vi "E3631A_Voltage Controller.vi"(5 "Channel Controller":T1(ring)=enum."Voltage 3", 6 "Voltage 3":dbl=-3.3 format="%.3g", 7 "Initialize":bool, 8 "error in (no error)":errorcluster, 9 "Voltage 2":dbl=3.3 format="%.3g", 10 "Voltage 1":dbl=3.3 format="%.3g", 11 "VISA resource name":refnum<visa-resource-name>="GPIB0::5::INSTR") -> (0 "error out":errorcluster, 3 "VISA resource name out":refnum<visa-resource-name>="GPIB0::5::INSTR")   [LabVIEW 2012]
uses:
  _Employee_Folders/Andy temp/All Driver/agilent/Agilent E363X Series/Agilent E363X Series.lvlib
panel:
  in  "Channel 3":i32(ring)=3 items=["Channel 1"=1, "Channel 2"=2, "Channel 3"=3]
  in  "Channel 2":i32(ring)=2 items=["Channel 1"=1, "Channel 2"=2, "Channel 3"=3]
  in  "Channel 1":i32(ring)=1 items=["Channel 1"=1, "Channel 2"=2, "Channel 3"=3]
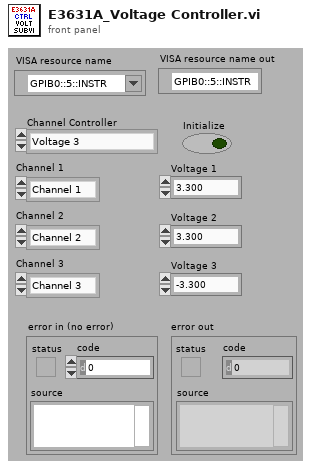
[diagram p1: front panel]
types:
  T1 = enum16{"Idle...", "Voltage 1", "Voltage 2", "Voltage 3"}
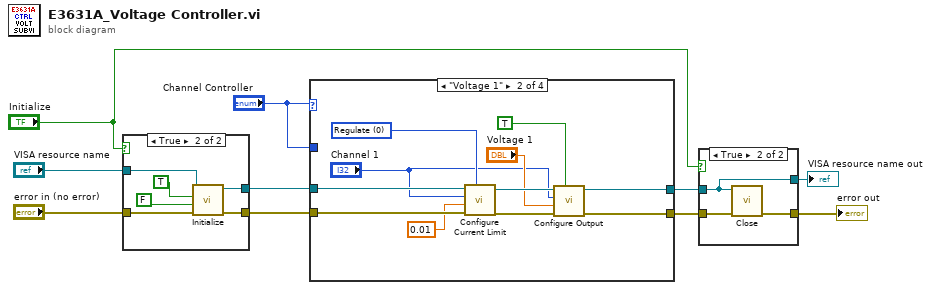
[diagram p0: block diagram]
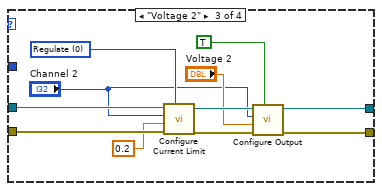
[diagram p5: hidden frame]
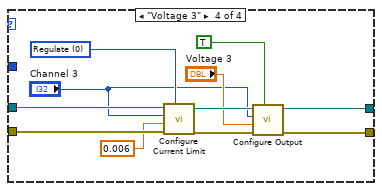
[diagram p6: hidden frame]
diagram:
  n1 = case shown="True" "Initialize" {
    tunnel: "error in (no error)" -> [w11 w18]
    tunnel: [w11 w17] -> w9
    tunnel: [w12 w16] -> w8
    tunnel: "VISA resource name" -> [w12 w13]
    frame False {
    }
    frame True {
      n2 = call "Initialize.vi"("error in (no error)"=w18, "Reset? (T: Yes)"=FALSE, "ID Query? (T: Yes)"=TRUE, "VISA resource name"=w13) -> ("error out"=w17:errorcluster, "VISA resource name out"=w16:refnum<visa-resource-name>)  [unwired: 6 in]
    }
  }
  n3 = case shown="\"Voltage 1\"" "Channel Controller" {
    tunnel: w9 -> [w19 w31 w42 w53]
    tunnel: w8 -> [w20 w30 w41 w52]
    tunnel: [w19 w24 w35 w46] -> w7
    tunnel: [w20 w23 w34 w45] -> w6
    tunnel: "Channel Controller" -> [_ _ _ _]
    frame "Idle...", Default {
    }
    frame "Voltage 1" {
      w28 = u16 0 items=["Regulate", "Trip"] ("Behavior (0: Regulate)")
      n4 = call "Configure Current Limit.vi"("Behavior (0: Regulate)"=w28, "error in (no error)"=w31, "Current Limit (0.0 A)"=0.01, "Channel (1: Channel 1)"="Channel 1", "VISA resource name"=w30) -> ("error out"=w26:errorcluster, "VISA resource name out"=w27:refnum<visa-resource-name>)  [unwired: 5 in]
      n5 = call "Configure Output.vi"("Enable Output (T: Enable)"=TRUE, "error in (no error)"=w26, "Voltage Level (0.0 V)"="Voltage 1", "Channel (1: Channel 1)"="Channel 1", "VISA resource name"=w27) -> ("error out"=w24:errorcluster, "VISA resource name out"=w23:refnum<visa-resource-name>)  [unwired: 5 in]
    }
    frame "Voltage 2" {
      w39 = u16 0 items=["Regulate", "Trip"] ("Behavior (0: Regulate)")
      n6 = call "Configure Current Limit.vi"("Behavior (0: Regulate)"=w39, "error in (no error)"=w42, "Current Limit (0.0 A)"=0.2, "Channel (1: Channel 1)"="Channel 2", "VISA resource name"=w41) -> ("error out"=w37:errorcluster, "VISA resource name out"=w38:refnum<visa-resource-name>)  [unwired: 5 in]
      n7 = call "Configure Output.vi"("Enable Output (T: Enable)"=TRUE, "error in (no error)"=w37, "Voltage Level (0.0 V)"="Voltage 2", "Channel (1: Channel 1)"="Channel 2", "VISA resource name"=w38) -> ("error out"=w35:errorcluster, "VISA resource name out"=w34:refnum<visa-resource-name>)  [unwired: 5 in]
    }
    frame "Voltage 3" {
      w50 = u16 0 items=["Regulate", "Trip"] ("Behavior (0: Regulate)")
      n8 = call "Configure Current Limit.vi"("Behavior (0: Regulate)"=w50, "error in (no error)"=w53, "Current Limit (0.0 A)"=0.006, "Channel (1: Channel 1)"="Channel 3", "VISA resource name"=w52) -> ("error out"=w48:errorcluster, "VISA resource name out"=w49:refnum<visa-resource-name>)  [unwired: 5 in]
      n9 = call "Configure Output.vi"("Enable Output (T: Enable)"=TRUE, "error in (no error)"=w48, "Voltage Level (0.0 V)"="Voltage 3", "Channel (1: Channel 1)"="Channel 3", "VISA resource name"=w49) -> ("error out"=w46:errorcluster, "VISA resource name out"=w45:refnum<visa-resource-name>)  [unwired: 5 in]
    }
  }
  n10 = case shown="True" "Initialize" {
    tunnel: w7 -> [w55 w58]
    tunnel: w6 -> [w54 w56]
    tunnel: [w55 w57] -> w5
    tunnel: [w54 w56] -> w1
    frame False {
    }
    frame True {
      n11 = call "Close.vi"("error in (no error)"=w58, "VISA resource name"=w56) -> ("error out"=w57:errorcluster)  [unwired: 9 in]
    }
  }
  "error out" <- w5
  "VISA resource name out" <- w1
